vi "Tophat Init LUT.vi"(7 "Number of  Elements":i32=80000, 8 "Df":i16=200, 9 "f0":i16=1350) -> (3 "Init Data Out":i16[](array[numeric]))   [LabVIEW 2016]
uses:
  <vilib>/Analysis/2dsp.llb/Inverse Real FFT.vi
  <vilib>/Analysis/NI_AALPro.lvlib
panel:
  out "f(t) half":i32[](graph)
  out "min value":i32=-32360
  out "max value":i32=-32768
  out "f(t)":i32[](graph)
  out "Frequency Domain Signal":i64[](graph)
  # "This is the max number of elements that will sit in a 16 bit wide block of memory"
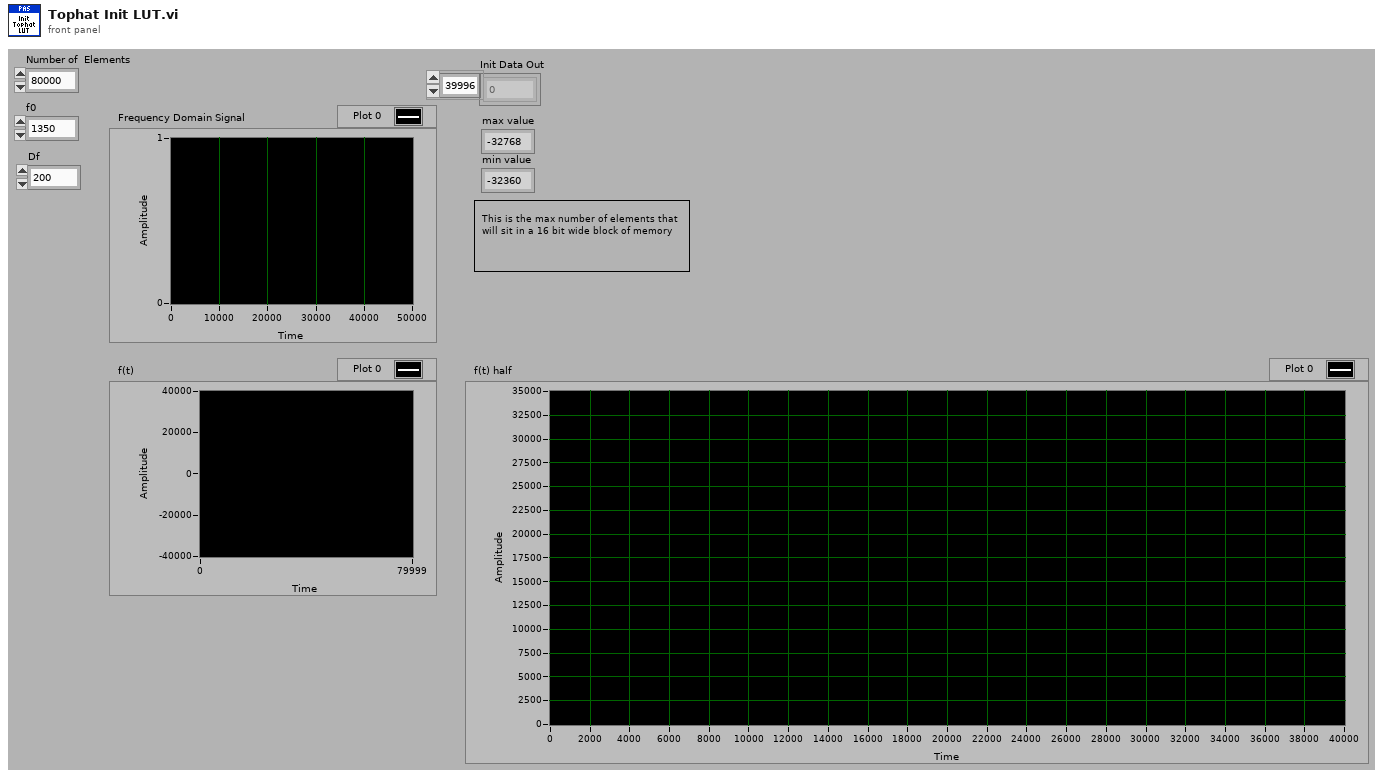
[diagram p1: front panel]
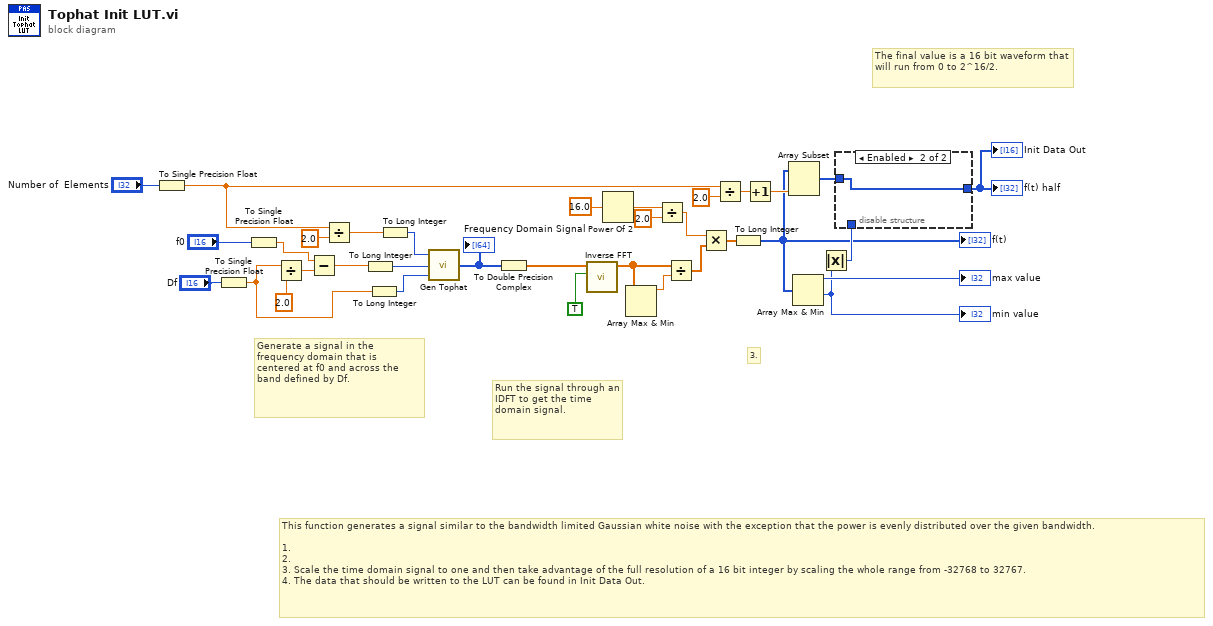
[diagram p0: block diagram]
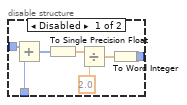
[diagram p2: hidden frame]
diagram:
  # "The final value is a 16 bit waveform that will run from 0 to 2^16/2."
  # "Generate a signal in the frequency domain that is centered at f0 and across the band defined by Df."
  # "3."
  # "Run the signal through an IDFT to get the time domain signal."
  # "This function generates a signal similar to the bandwidth limited Gaussian white noise with the exception that the power is evenly distributed over the given bandwidth.\n\n1. \n2. \n3. Scale the time domain signal to one and then take advantage of the full resolution of a 16 bit integer by scaling the whole range from -32768 to 32767.\n4. The data that should be written to the LUT can be found in Init Data Out."
  n1 = To Single Precision Float(number="Number of  Elements") -> (single precision float=w9:sgl)
  n2 = To Single Precision Float(number="Df") -> (single precision float=w4:sgl)
  n3 = To Single Precision Float(number="f0") -> (single precision float=w11:sgl)
  n4 = Divide(x=w4, y=sgl 2.0) -> (x/y=w26:sgl)
  n5 = Subtract(x=w11, y=w26) -> (x-y=w6:sgl)
  n6 = Divide(x=w9, y=sgl 2.0) -> (x/y=w8:sgl)
  n7 = To Long Integer(number=w6) -> (32bit integer=w5:i32)
  n8 = To Long Integer(number=w4) -> (32bit integer=w3:i32)
  n9 = To Long Integer(number=w8) -> (32bit integer=w7:i32)
  n10 = call "Gen Tophat.vi"("Frequency Span"=w3, "Lower Frequency \nLocation"=w5, "Nyquist Frequency\nLocation"=w7) -> ("Waveform Graph"=w2:i64[])
  "Frequency Domain Signal" <- w2
  n11 = To Double Precision Complex(1:w2) -> (0:w1:cdb[])
  n12 = call-poly <vilib>:"Inverse FFT.vi"("shift?"=TRUE, "FFT {X}"=w1) -> ("X"=w30:dbl[])  [unwired: 9 out]
  n13 = Power Of 2(x=sgl 16.0) -> (2^x=w29:sgl)
  n14 = Array Max & Min(array=w30) -> (max value=w20:dbl)  [unwired: 3 out]
  n15 = Divide(x=w29, y=sgl 2.0) -> (x/y=w27:sgl)
  n16 = Divide(x=w30, y=w20) -> (x/y=w21:dbl[])
  n17 = Multiply(x=w27, y=w21) -> (x*y=w15:dbl[])
  n18 = Divide(x=w9, y=sgl 2.0) -> (x/y=w23:sgl)
  n19 = To Long Integer(number=w15) -> (32bit integer=w14:i32[])
  "f(t)" <- w14
  n20 = Increment(x=w23) -> (x+1=w22:sgl)
  n21 = Array Subset(array=w14, length=w22) -> (w19:i32[])  [unwired: 1 in]
  n22 = Array Max & Min(array=w14) -> (max value=→"max value":i32, min value=w17:i32)  [unwired: 2 out]
  "min value" <- w17
  n23 = Absolute Value(x=w17) -> (abs(x)=w16:i32)
  n24 = disable-structure shown="Enabled" {
    disable-tunnel: w19 -> [w41 w42]
    disable-tunnel: [w38 w42] -> w18
    disable-tunnel: w16 -> [w37 _]
    frame Disabled {
      n25 = Add(x=w41, y=w37) -> (x+y=w36:i32[])
      n26 = To Single Precision Float(number=w36) -> (single precision float=w35:sgl[])
      n27 = Divide(x=w35, y=sgl 2.0) -> (x/y=w39:sgl[])
      n28 = To Word Integer(number=w39) -> (16bit integer=w38:i16[])
    }
    frame Enabled {
    }
  }
  "Init Data Out" <- w18
  "f(t) half" <- w18
